vi "FrequencyDomainCorrelationImages.vi"(10 "Template":T1, 11 "Image":T1) -> (3 "FDCorrelation":sgl[][](array[numeric]) format="%.2f")   [LabVIEW 2014]
uses:
  <vilib>/vision/Image Controls.llb/IMAQ Image.ctl
  <vilib>/vision/NI_Vision_Development_Module.lvlib
panel:
  out "Image Dst Out 2":T1(plugin-control)
  out "Image Dst Out":T1(plugin-control)
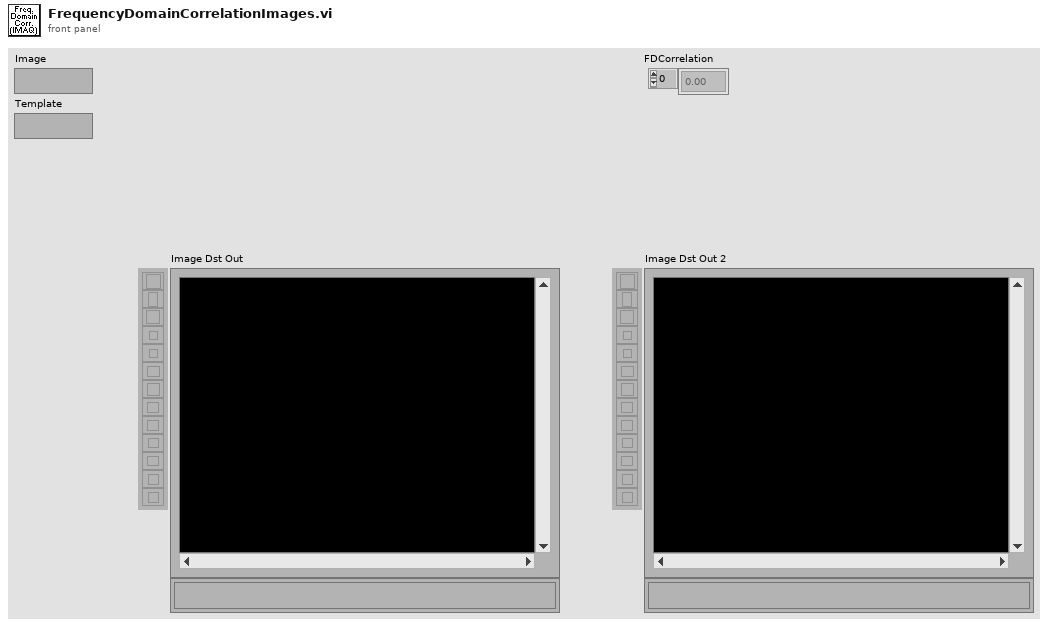
[diagram p1: front panel]
types:
  T1 = typedef "IMAQ Image.ctl" = refnum<image>
  T2 = enum16{"Full", "Left-Top", "Top-Right", "Right-Bottom", "Bottom-Left", "Left", "Top", "Right", "Bottom"}
  T3 = typedef "Image Type" = u32
  T4 = enum32{"Real", "Imaginary", "Magnitude", "Phase"}
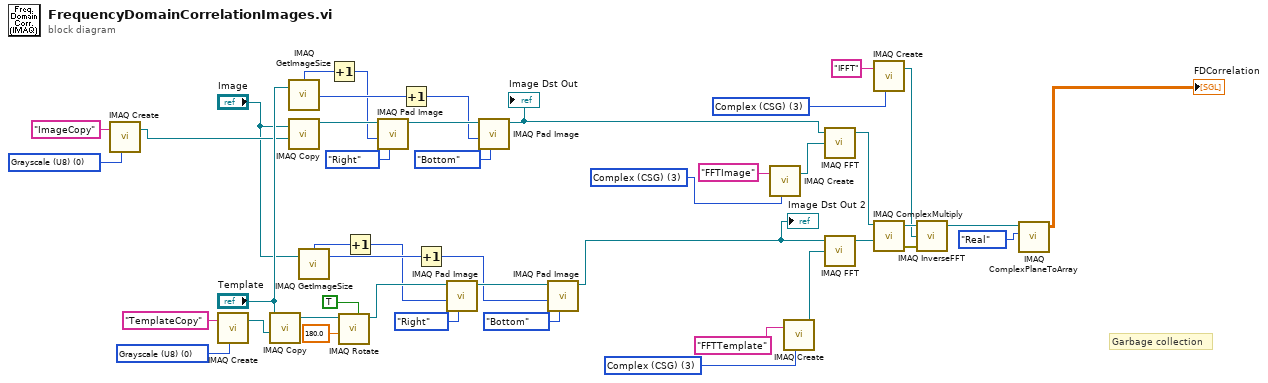
[diagram p0: block diagram]
diagram:
  w30 = T3 0 items=["Grayscale (U8)", "Grayscale (I16)", "Grayscale (SGL)", "Complex (CSG)", "RGB (U32)", "HSL (U32)", "RGB (U64)", "Grayscale (U16)"] ("Image Type")
  w32 = T3 0 items=["Grayscale (U8)", "Grayscale (I16)", "Grayscale (SGL)", "Complex (CSG)", "RGB (U32)", "HSL (U32)", "RGB (U64)", "Grayscale (U16)"] ("Image Type")
  w36 = T3 3 items=["Grayscale (U8)", "Grayscale (I16)", "Grayscale (SGL)", "Complex (CSG)", "RGB (U32)", "HSL (U32)", "RGB (U64)", "Grayscale (U16)"] ("Image Type")
  w42 = T3 3 items=["Grayscale (U8)", "Grayscale (I16)", "Grayscale (SGL)", "Complex (CSG)", "RGB (U32)", "HSL (U32)", "RGB (U64)", "Grayscale (U16)"] ("Image Type")
  w44 = T3 3 items=["Grayscale (U8)", "Grayscale (I16)", "Grayscale (SGL)", "Complex (CSG)", "RGB (U32)", "HSL (U32)", "RGB (U64)", "Grayscale (U16)"] ("Image Type")
  # "Garbage collection"
  n1 = call "IMAQ Create"("Image Name"="ImageCopy", "Image Type"=w30) -> ("New Image"=w23:T1)  [unwired: 3 in, 1 out]
  n2 = call "IMAQ Create"("Image Name"="TemplateCopy", "Image Type"=w32) -> ("New Image"=w29:T1)  [unwired: 3 in, 1 out]
  n3 = call "IMAQ Copy"("Image Dst"=w29, "Image Src"="Template") -> ("Image Dst Out"=w20:T1)  [unwired: 4 in, 1 out]
  n4 = call "IMAQ GetImageSize"("Image"="Template") -> ("Y Resolution"=w14:i32, "X Resolution"=w17:i32)  [unwired: 3 in, 1 out]
  n5 = call "IMAQ Copy"("Image Dst"=w23, "Image Src"="Image") -> ("Image Dst Out"=w22:T1)  [unwired: 4 in, 1 out]
  n6 = call "IMAQ GetImageSize"("Image"="Image") -> ("Y Resolution"=w5:i32, "X Resolution"=w6:i32)  [unwired: 3 in, 1 out]
  n7 = Increment(x=w17) -> (x+1=w1:i32)
  n8 = call "IMAQ Rotate"("Maintain Size"=TRUE, "Angle (degrees)"=sgl 180.0, "Image Src"=w20) -> ("Image Dst Out"=w9:T1)  [unwired: 7 in, 1 out]
  n9 = Increment(x=w6) -> (x+1=w3:i32)
  n10 = call "IMAQ Pad Image.vi"("Padding Type"=T2."Right", "Pixels"=w1, "Image Src"=w22) -> ("Image Dest Out"=w15:T1)  [unwired: 8 in]
  n11 = Increment(x=w14) -> (x+1=w2:i32)
  n12 = Increment(x=w5) -> (x+1=w4:i32)
  n13 = call "IMAQ Pad Image.vi"("Padding Type"=T2."Right", "Pixels"=w3, "Image Src"=w9) -> ("Image Dest Out"=w8:T1)  [unwired: 8 in]
  n14 = call "IMAQ Pad Image.vi"("Padding Type"=T2."Bottom", "Pixels"=w2, "Image Src"=w15) -> ("Image Dest Out"=w13:T1)  [unwired: 8 in]
  "Image Dst Out" <- w13
  n15 = call "IMAQ Pad Image.vi"("Padding Type"=T2."Bottom", "Pixels"=w4, "Image Src"=w8) -> ("Image Dest Out"=w7:T1)  [unwired: 8 in]
  "Image Dst Out 2" <- w7
  n16 = call "IMAQ Create"("Image Name"="FFTImage", "Image Type"=w44) -> ("New Image"=w41:T1)  [unwired: 3 in, 1 out]
  n17 = call "IMAQ Create"("Image Name"="FFTTemplate", "Image Type"=w36) -> ("New Image"=w25:T1)  [unwired: 3 in, 1 out]
  n18 = call "IMAQ FFT"("Image Dst"=w41, "Image Src"=w13) -> ("Image Dst Out"=w27:T1)  [unwired: 2 in, 1 out]
  n19 = call "IMAQ FFT"("Image Dst"=w25, "Image Src"=w7) -> ("Image Dst Out"=w35:T1)  [unwired: 2 in, 1 out]
  n20 = call "IMAQ Create"("Image Name"="IFFT", "Image Type"=w42) -> ("New Image"=w26:T1)  [unwired: 3 in, 1 out]
  n21 = call "IMAQ ComplexMultiply"("Image Src A"=w27, "Image Src B"=w35) -> ("Image Dst Out"=w39:T1, "error out"=w40:errorcluster)  [unwired: 5 in]
  n22 = call "IMAQ InverseFFT"("error in (no error)"=w40, "Image Dst"=w26, "Image Src"=w39) -> ("Image Dst Out"=w34:T1)  [unwired: 1 in, 1 out]
  n23 = call "IMAQ ComplexPlaneToArray"("Plane"=T4."Real", "Image"=w34) -> ("Image Pixels (float)"=→"FDCorrelation":sgl[][])  [unwired: 3 in, 1 out]
